vi "Check Image Matches Design.vi"(8 "error in":errorcluster, 10 "board image":T2, 11 "board in":refnum<class "Board Design.lvclass">) -> (0 "error out":errorcluster, 2 "pass?":T1, 3 "board out":refnum<class "Board Design.lvclass">)   [LabVIEW 2023, in "Board Design.lvclass"]
doc: "Check the board image and determine if it matches the expected appearance."
uses:
  Board Design.lvclass
  Common/Board Image.ctl
  Common/Pass Fail Boolean.ctl
  Component/Component.lvclass
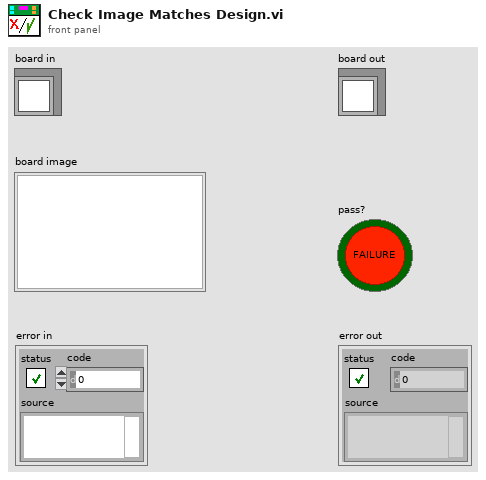
[diagram p1: front panel]
types:
  T1 = typedef "Pass Fail Boolean.ctl" = bool
  T2 = typedef "Board Image.ctl" = picture
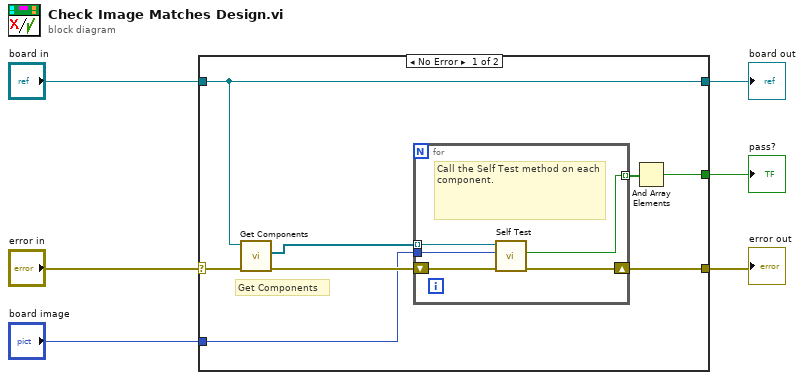
[diagram p0: block diagram]
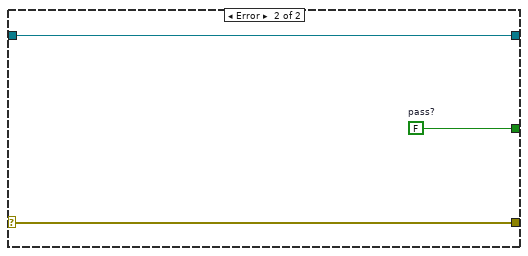
[diagram p2: hidden frame]
diagram:
  n1 = case shown="No Error" "error in" {
    selector: "error in" -> [w11 w22]
    tunnel: [w14 w22] -> w5
    tunnel: [w9 w20] -> w3
    tunnel: "board in" -> [w9 w20]
    tunnel: [w12 w21] -> w2
    tunnel: "board image" -> [w7 _]
    frame No Error {
      # "Get Components"
      n2 = call-dynamic "Get Components.vi"("error in"=w11, "board in"=w9) -> ("error out"=w10:errorcluster, "components"=w13:refnum<class "Component.lvclass">[])  [unwired: 7 in, 1 out]
      n3 = for {
        tunnel: w13 -> [w16] mode=indexing
        tunnel: [w19] -> w8 mode=indexing
        shift-right: [w18] -> w14
        shift-left: w10 -> [w17]
        tunnel: w7 -> [w15]
        # "Call the Self Test method on each component."
        n4 = call-dynamic "Self Test.vi"("error in"=w17, "Board Image"=w15, "Component in"=w16) -> ("error out"=w18:errorcluster, "Pass?"=w19:T1)  [unwired: 6 in, 1 out]
      }
      n5 = And Array Elements(Boolean array=w8) -> (logical AND=w12:bool)
    }
    frame Error {
      w21 = T1 FALSE  # pass?
    }
  }
  "error out" <- w5
  "board out" <- w3
  "pass?" <- w2
